vi "PH_Beckhoff.handle Analog Inputs.vi"(0 "i ref in":refnum<vi>, 1 "Old Values":T1, 2 "Current Analog Inputs":u32[](array[numeric]), 3 "Quality":bool, 4 "Difference to handle an analog input as change":u32=1, 5 "error in":errorcluster) -> (14 "i ref out":refnum<vi>, 17 "#s of changed analog Inputs":i32[](array[numeric]), 19 "error out":errorcluster)   [LabVIEW 2014, in "PH_Beckhoff.lvlib"]
doc: "This VI handles the incoming information about analog inputs: if value or quality changed, these are set to own attributes and the scaled information is published via DIM."
uses:
  PH_Beckhoff.lvlib
  PH_Beckhoff.Values.ctl
  PH_Beckhoff.Sonderklemmen Inputs.ctl
  PH_Beckhoff.Analog Inputs.ctl
  PH_Beckhoff.Scaling Type.ctl
  PH_Beckhoff.Analog Outputs.ctl
  PH_Beckhoff.Digital Inputs.ctl
  PH_Beckhoff.Digital Outputs.ctl
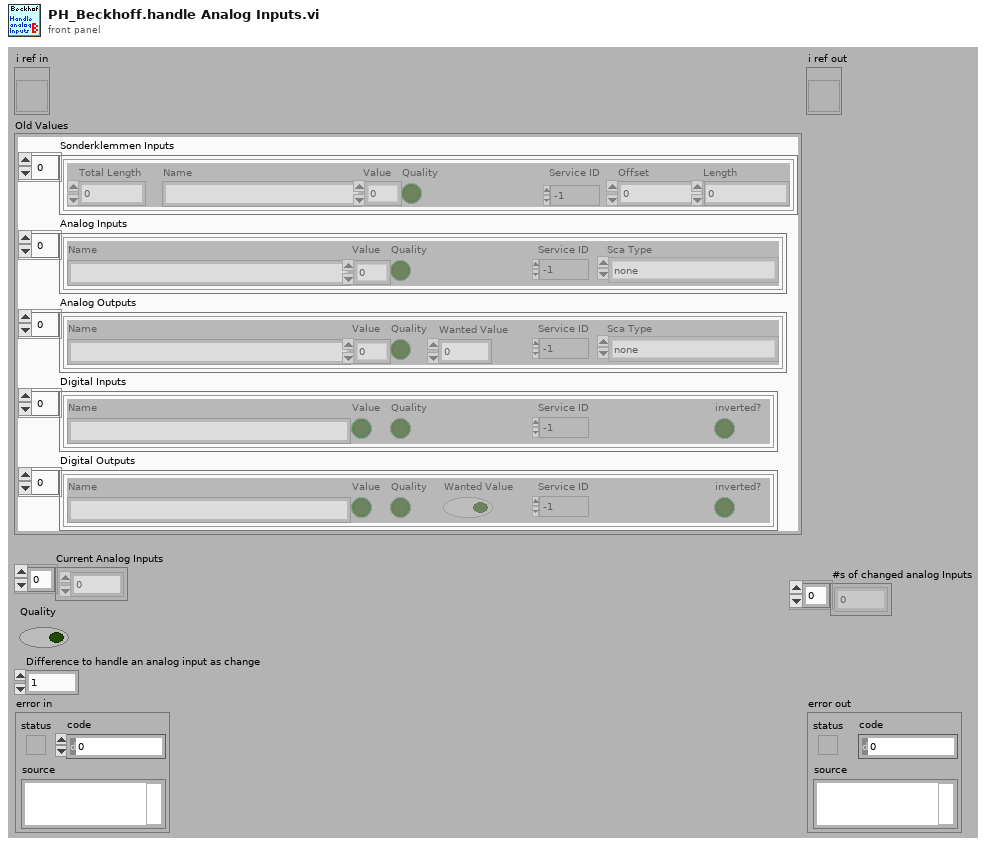
[diagram p1: front panel]
types:
  T1 = typedef "PH_Beckhoff.lvlib/PH_Beckhoff.Values.ctl" = cluster{"Sonderklemmen Inputs":T2, "Analog Inputs":T3, "Analog Outputs":T5, "Digital Inputs":T6, "Digital Outputs":T7}
  T2 = typedef "PH_Beckhoff.lvlib/PH_Beckhoff.Sonderklemmen Inputs.ctl" = cluster{"Total Length":u32, "Name":string, "Value":u64, "Quality":bool, "Service ID":i32, "Offset":u32, "Length":u32}[]
  T3 = typedef "PH_Beckhoff.lvlib/PH_Beckhoff.Analog Inputs.ctl" = cluster{"Name":string, "Value":u32, "Quality":bool, "Service ID":i32, "Sca Type":T4}[]
  T4 = typedef "PH_Beckhoff.lvlib/PH_Beckhoff.Scaling Type.ctl" = enum16{"none", "0 ... 15 Bit -> 0 ... 5", "0 ... 15 Bit -> 0 ... 10", "0 ... 15 Bit -> 0 ... 25", "0 ... 15 Bit -> 4 ... 20", "0 ... 15 Bit -> 0 ... 1", "0 ... 15 Bit -> 0 ... 20000", "0 ... 15 Bit -> 0 ... 24000"}
  T5 = typedef "PH_Beckhoff.lvlib/PH_Beckhoff.Analog Outputs.ctl" = cluster{"Name":string, "Value":u32, "Quality":bool, "Wanted Value":u32, "Service ID":i32, "Sca Type":T4}[]
  T6 = typedef "PH_Beckhoff.lvlib/PH_Beckhoff.Digital Inputs.ctl" = cluster{"Name":string, "Value":bool, "Quality":bool, "Service ID":i32, "inverted?":bool}[]
  T7 = typedef "PH_Beckhoff.lvlib/PH_Beckhoff.Digital Outputs.ctl" = cluster{"Name":string, "Value":bool, "Quality":bool, "Wanted Value":bool, "Service ID":i32, "inverted?":bool}[]
  T8 = typedef "PH_Beckhoff.lvlib/PH_Beckhoff.i attribute.ctl" = cluster{"GUI Refs":T9, "operation?":bool, "Default Prdc Interval":i32, "Connection":T10, "AMS Net ID":T11, "Klemmencluster: # of":T12, "Values":T1, "IP":string, "Description":string, "configured?":bool, "Change Manager":cluster{"Detemination wanted?":bool, "Values changed at":cluster{"Sonderklemmen Inputs":i32[], "Analog Inputs":i32[], "Analog Outputs":i32[], "Digital Inputs":i32[], "Digital Outputs":i32[]}}, "Difference to handle an analog input as change":u32}
  T9 = typedef "PH_Beckhoff.lvlib/PH_Beckhoff.GUI Refs.ctl" = cluster{"ADS Error":refnum<vi>, "Values":refnum<vi>, "configured?":refnum<vi>, "Connection":refnum<vi>, "IP":refnum<vi>, "Prdc Int [ms]":refnum<vi>}
  T10 = typedef "PH_Beckhoff.lvlib/PH_Beckhoff.Connectivity.ctl" = cluster{"DLL?":bool, "Port?":bool, "Client?":bool, "Ping?":bool, "unsuccessful Pings":u32}
  T11 = typedef "Beckhoff - Driver np.lvlib/Beckhoff Access.ctl" = cluster{"DLL path":path, "AMS Net ID":cluster{"1st # of IP":u8, "2nd # of IP":u8, "3rd # of IP":u8, "4th # of IP":u8, "In Port":u8, "Out Port":u8}}
  T12 = typedef "Beckhoff - Driver np.lvlib/Klemmendeclarer.ctl" = cluster{"Offset due to Sonderklemms":u32, "analog Inputs":u32, "analog Outputs":u32, "digital Input Bits":u32, "digital Output Bits":u32}
  T13 = cluster{"Name":string, "Value":u32, "Quality":bool, "Service ID":i32, "Sca Type":T4}
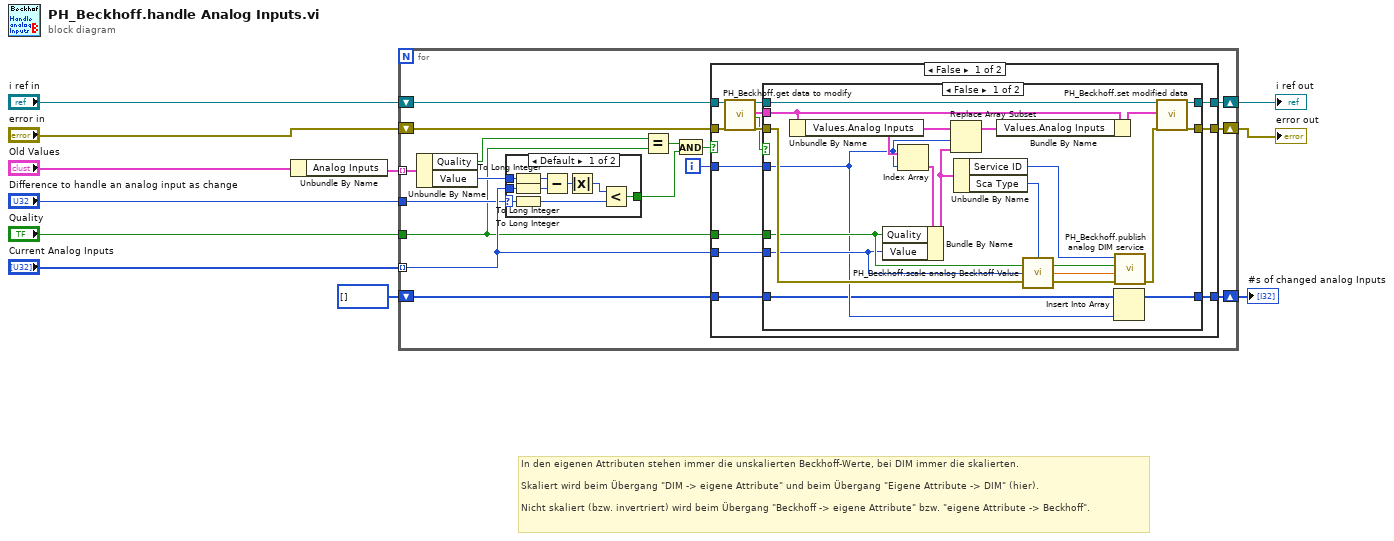
[diagram p0: block diagram]
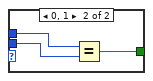
[diagram p2: hidden frame]
diagram:
  # "In den eigenen Attributen stehen immer die unskalierten Beckhoff-Werte, bei DIM immer die skalierten.\n\nSkaliert wird beim Übergang \"DIM -> eigene Attribute\" und beim Übergang \"Eigene Attribute -> DIM\" (hier).\n\nNicht skaliert (bzw. invertriert) wird beim Übergang \"Beckhoff -> eigene Attribute\" bzw. \"eigene Attribute -> Beckhoff\"."
  n1 = Unbundle By Name("Old Values") -> ("Analog Inputs"=w11:T3)
  n2 = for {
    tunnel: w11 -> [w27] mode=indexing
    tunnel: "Quality" -> [w13]
    tunnel: "Current Analog Inputs" -> [w15] mode=indexing
    shift-right: [w22] -> w7
    shift-left: "error in" -> [w23]
    shift-right: [w20] -> w8
    shift-left: "i ref in" -> [w21]
    shift-right: [w18] -> w3
    shift-left: i32[] [] ("Array") -> [w17]
    tunnel: "Difference to handle an analog input as change" -> [w14]
    i -> [w19]
    n3 = Unbundle By Name(w27) -> ("Quality"=w12:bool, "Value"=w16:u32)
    n4 = case shown="Default" w14 {
      selector: w14 -> [w30 _]
      tunnel: [w29 w39] -> w25
      tunnel: w16 -> [w35 w38]
      tunnel: w15 -> [w36 w37]
      frame Default {
        n5 = To Long Integer(number=w35) -> (32bit integer=w33:i32)
        n6 = To Long Integer(number=w36) -> (32bit integer=w32:i32)
        n7 = To Long Integer(number=w30) -> (32bit integer=w28:i32)
        n8 = Subtract(x=w33, y=w32) -> (x-y=w34:i32)
        n9 = Absolute Value(x=w34) -> (abs(x)=w31:i32)
        n10 = Less?(x=w31, y=w28) -> (x < y?=w29:bool)
      }
      frame 0, 1 {
        n11 = Equal?(x=w38, y=w37) -> (x = y?=w39:bool)
      }
    }
    n12 = Equal?(x=w12, y=w13) -> (x = y?=w26:bool)
    n13 = And(x=w26, y=w25) -> (x .and. y?=w24:bool)
    n14 = case shown="False" w24 {
      tunnel: w23 -> [w52 w77]
      tunnel: [w50 w77] -> w22
      tunnel: w21 -> [w49 w76]
      tunnel: [w47 w76] -> w20
      tunnel: w19 -> [w44 _]
      tunnel: w13 -> [w43 _]
      tunnel: w15 -> [w42 _]
      tunnel: [w41 w75] -> w18
      tunnel: w17 -> [w40 w75]
      frame False {
        n15 = call "PH_Beckhoff.get data to modify.vi"("i ref in"=w49, "error in (no error)"=w52) -> ("i ref out"=w48:refnum<vi>, "i attribute"=w45:T8, "timed out"=w46:bool, "error out"=w51:errorcluster)  [unwired: 14 in]
        n16 = case shown="False" w46 {
          tunnel: w51 -> [w59 w73]
          tunnel: [w71 w73] -> w50
          tunnel: w48 -> [w70 w74]
          tunnel: [w69 w74] -> w47
          tunnel: w45 -> [w67 _]
          tunnel: w44 -> [w54 _]
          tunnel: w43 -> [w57 _]
          tunnel: w42 -> [w56 _]
          tunnel: [w55 w72] -> w41
          tunnel: w40 -> [w53 w72]
          frame False {
            n17 = Unbundle By Name(w67) -> ("Values.Analog Inputs"=w65:T3)
            n18 = Index Array(array=w65, index=w54) -> (element=w64:T13)
            n19 = Bundle By Name(cluster=w64, "Quality"=w57, "Value"=w56) -> (w58:T13)
            n20 = Replace Array Subset(array=w65, new element=w58, index=w54) -> (w66:T3)
            n21 = Unbundle By Name(w58) -> ("Service ID"=w62:i32, "Sca Type"=w61:T4)
            n22 = Bundle By Name(cluster=w67, "Values.Analog Inputs"=w66) -> (w68:T8)
            n23 = call "PH_Beckhoff.scale analog Beckhoff Value.vi"("Beckhoff value"=w56, "Scaling Type"=w61) -> ("DIM value"=w60:dbl)
            n24 = Insert Into Array(array=w53, new element=w54) -> (w55:i32[])  [unwired: 1 in]
            n25 = call "PH_Beckhoff.publish analog DIM service.vi"("error in"=w59, "Value"=w60, "Quality ok?"=w57, "Service ID"=w62) -> ("error out"=w63:errorcluster)  [unwired: 4 in]
            n26 = call "PH_Beckhoff.set modified data.vi"("i ref in"=w70, "i attribute"=w68, "error in (no error)"=w63) -> ("i ref out"=w69:refnum<vi>, "error out"=w71:errorcluster)  [unwired: 15 in]
          }
          frame True {
          }
        }
      }
      frame True {
      }
    }
  }
  "i ref out" <- w8
  "error out" <- w7
  "#s of changed analog Inputs" <- w3
